vi "FlatToRichniswitch_grpc_GetAttributeViStringResponse.vi"(5 "OutputClusterType":T1, 11 "InputCluster":T2) -> (3 "OutputCluster":T1)   [LabVIEW 2021, in "NI Switch_client.lvlib"]
uses:
  NI Switch_client.lvlib
  niswitch_grpc_GetAttributeViStringResponse_Flat.ctl
  niswitch_grpc_GetAttributeViStringResponse.ctl
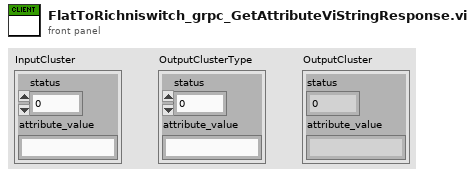
[diagram p1: front panel]
types:
  T1 = typedef "NI Switch_client.lvlib/niswitch_grpc_GetAttributeViStringResponse.ctl" = cluster{"status":i32, "attribute_value":string}
  T2 = typedef "NI Switch_client.lvlib/niswitch_grpc_GetAttributeViStringResponse_Flat.ctl" = cluster{"status":i32, "attribute_value":string}
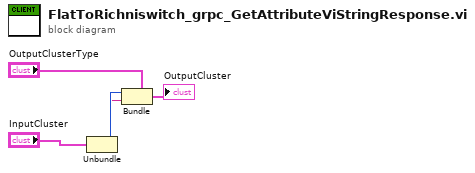
[diagram p0: block diagram]
diagram:
  n1 = Unbundle "Unbundle"("InputCluster") -> ("status"=w2:i32, "attribute_value"=w1:string)
  n2 = Bundle "Bundle"(cluster="OutputClusterType", "status"=w2, "attribute_value"=w1) -> (→"OutputCluster":T1)
